vi "Gui_Set_Laser_Refs.vi"(0 "Laser Refs":refnum<vi>[](array[refnum]), 1 "EXPERIMENT Inputs":T1={"Setup"="", "Date"="", "User Name"="", "Comment"="", "Experiment Procedures"=[], "Chemical Source"="", "Sample Components"=[], "Species"=[], "Laser 1"={"Used"=TRUE, "Name"="Spectroscopy", "Wavelength"=1000.0, "Energy"=25.0}, "Laser 2"={"Used"=TRUE, "Name"="Spectroscopy", "Wavelength"=1000.0, "Energy"=25.0}, "Laser 3"={"Used"=TRUE, "Name"="Spectroscopy", "Wavelength"=1000.0, "Energy"=25.0}, "Laser 4"={"Used"=TRUE, "Name"="Spectroscopy", "Wavelength"=1000.0, "Energy"=25.0}, "Laser 5"={"Used"=TRUE, "Name"="Spectroscopy", "Wavelength"=1000.0, "Energy"=25.0}, "Lamp 1"={"Used"=TRUE, "Name"="Spectroscopy", "Wavelength"=1000.0, "Attenuation"=25.0}, "Lamp 2"={"Used"=TRUE, "Name"="Spectroscopy", "Wavelength"=1000.0, "Attenuation"=25.0}, "Gas 1"={"Used"=TRUE, "Name"="Spectroscopy", "Pressure"=1000.0}, "Gas 2"={"Used"=TRUE, "Name"="Spectroscopy", "Pressure"=1000.0}, "Gas 3"={"Used"=TRUE, "Name"="Spectroscopy", "Pressure"=1000.0}, "Gas 4"={"Used"=TRUE, "Name"="Spectroscopy", "Pressure"=1000.0}, "Gas 5"={"Used"=TRUE, "Name"="Spectroscopy", "Pressure"=1000.0}}, 2 "Path":path, 3 "error in (no error)":errorcluster) -> (7 "Laser Refs out":refnum<vi>[](array[refnum]), 10 "error out":errorcluster caption="sortie d'erreur")   [LabVIEW 2020]
doc: "This VI fills all the Laser ring lists with values read from a text file.\nA table of references to the Laser cluster controls is used."
uses:
  controls/EXPERIMENT_Inputs.ctl
  controls/LASER_Inputs.ctl
  controls/LAMP_Inputs.ctl
  controls/GAS_Inputs.ctl
panel:
  # "Lasers"
  # "nm"
  # "mJ"
  # "Lamps"
  # "nm"
  # "dB"
  # "Gas"
  # "bar"
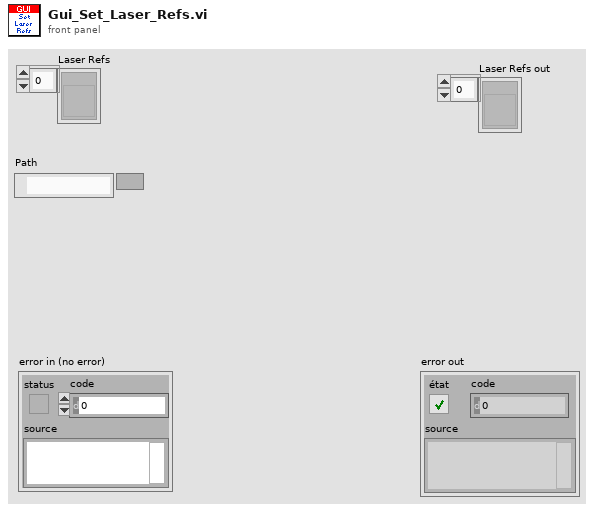
[diagram p1: front panel]
types:
  T1 = typedef "EXPERIMENT_Inputs.ctl" = cluster{"Setup":string, "Date":string, "User Name":string, "Comment":string, "Experiment Procedures":string[], "Chemical Source":string, "Sample Components":string[], "Species":string[], "Laser 1":T2, "Laser 2":T2, "Laser 3":T2, "Laser 4":T2, "Laser 5":T2, "Lamp 1":T3, "Lamp 2":T3, "Gas 1":T4, "Gas 2":T4, "Gas 3":T4, "Gas 4":T4, "Gas 5":T4}
  T2 = typedef "LASER_Inputs.ctl" = cluster{"Used":bool, "Name":string, "Wavelength":dbl, "Energy":dbl}
  T3 = typedef "LAMP_Inputs.ctl" = cluster{"Used":bool, "Name":string, "Wavelength":dbl, "Attenuation":dbl}
  T4 = typedef "GAS_Inputs.ctl" = cluster{"Used":bool, "Name":string, "Pressure":dbl}
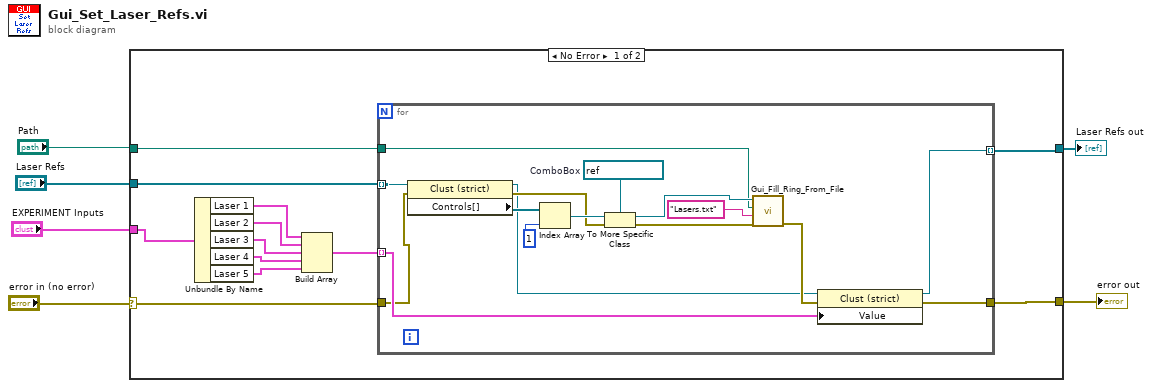
[diagram p0: block diagram]
diagram:
  n1 = case shown="No Error" "error in (no error)" {
    selector: "error in (no error)" -> [w18 w36]
    tunnel: [w9 w36] -> w6
    tunnel: "Laser Refs" -> [w11 w35]
    tunnel: [w10 w35] -> w3
    tunnel: "Path" -> [w8 _]
    tunnel: "EXPERIMENT Inputs" -> [w7 _]
    frame No Error {
      n2 = Unbundle By Name(w7) -> ("Laser 1"=w13:T2, "Laser 2"=w14:T2, "Laser 3"=w15:T2, "Laser 4"=w16:T2, "Laser 5"=w17:T2)
      n3 = Build Array(w13, w14, w15, w16, w17) -> (w12:T2[])
      n4 = for {
        tunnel: w12 -> [w34] mode=indexing
        tunnel: w11 -> [w25] mode=indexing
        tunnel: [w33] -> w10 mode=indexing
        tunnel: w18 -> [w24]
        tunnel: [w32] -> w9
        tunnel: w8 -> [w22]
        w26 = refnum<vi> refnum  # ComboBox
        n5 = property class="Clust (strict)"(reference=w25, error in=w24) -> (reference out=w20:refnum<vi>, error out=w23:errorcluster, "Controls[]"=w30:refnum<vi>[])
        n6 = Index Array(array=w30, index=1 ("indice")) -> (element=w28:refnum<vi>)
        n7 = To More Specific Class(target class=w26, reference=w28, error in=w23) -> (specific class reference=w27:refnum<vi>, error out=w19:errorcluster)
        n8 = call "Gui_Fill_Ring_From_File.vi"("error in (no error)"=w19, "Resource Name"="Lasers.txt", "Resource Path"=w22, "Refnum ChneDér"=w27) -> ("error out"=w21:errorcluster)  [unwired: 4 in, 3 out]
        n9 = property class="Clust (strict)"(reference=w20, error in=w21, "Value"=w34) -> (reference out=w33:refnum<vi>, error out=w32:errorcluster)
      }
    }
    frame Error {
    }
  }
  "error out" <- w6
  "Laser Refs out" <- w3
